vi "UI-BaseParamSet - 副本.vi"(8 "error in (no error)":errorcluster caption="错误输入（无错误）") -> (0 "error out":errorcluster caption="错误输出")   [LabVIEW 2017]
uses:
  Picture/SaveButtom.ctl
  Global System.vi
panel:
  in  "实际孔径":dbl
  in  "Program Update":bool
  in  "Machine Paramter Save Buttom":T1
  out "system time":string
  in  "选项卡控件":enum32{"BaseParamSet", "OtherParamSet"}(tab)
  in  "条码扫描周期":string
  in  "OUT Stack Weigh DataBits":string
  in  "OUT Stack Weigh BaudRate":string
  in  "OUT Stack Weigh VISA Name":refnum<visa-resource-name>="COM1"
  in  "OUT Stack Barcode DataBits":string
  in  "OUT Stack Barcode BaudRate":string
  in  "OUT Stack Barcode VISA Name":refnum<visa-resource-name>="COM1"
  in  "IN Stack Weigh DataBits":string
  in  "IN Stack Weigh BaudRate":string
  in  "IN Stack Weigh VISA Name":refnum<visa-resource-name>="COM1"
  in  "IN Stack Barcode DataBits":string
  in  "IN Stack Barcode BaudRate":string
  in  "IN Stack Barcode VISA Name":refnum<visa-resource-name>="COM1"
  in  "LoadProgram":string(combo)
  in  "BaseParams Save Buttom":T1
  in  "参数B":string
  in  "参数K":string
  in  "校正像素值":string
  in  "Tolerance Params Save":T1
  in  "单位距离":string
  # "秒"
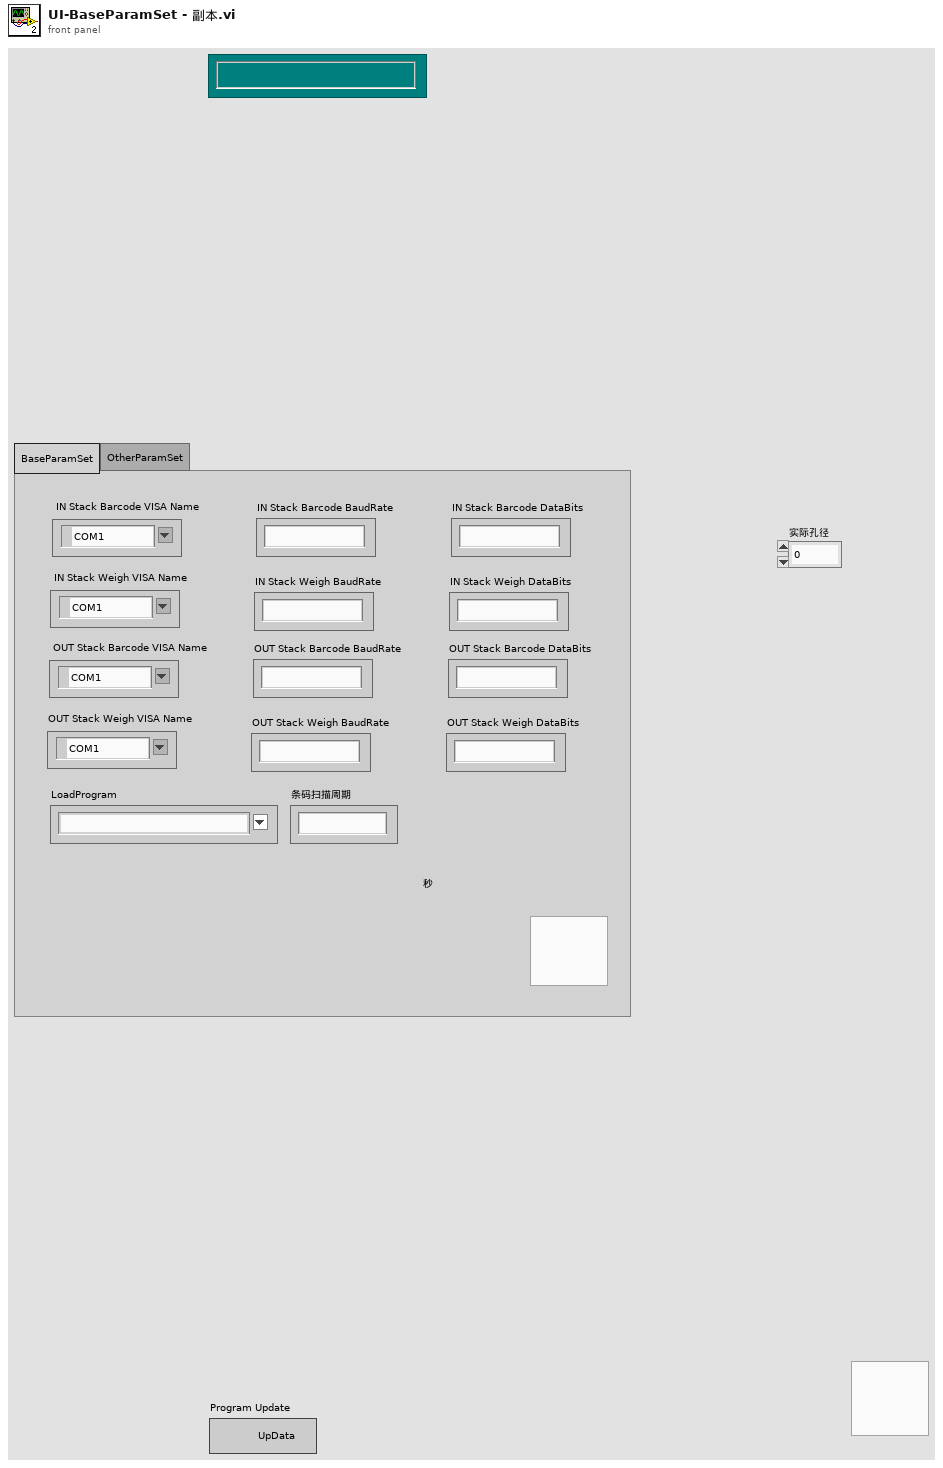
[diagram p1: front panel]
types:
  T1 = typedef "SaveButtom.ctl" = bool
  T2 = cluster{"master data":string, "priority":u16, "secondary data":string[]}
  T3 = cluster{"case name":string[], "queue array":refnum<queue>[]}
  T4 = cluster{"导通气缸上位置":bool, "导通气缸下位置\n":bool, "工位一料到位信号":bool, "工位二料到位信号":bool, "工位三料到位信号":bool, "转盘到位信号":bool, "凸轮感应信号":bool, "导通信号":bool, "真空":bool, "备用":bool, "备用":bool, "备用":bool, "备用":bool, "备用":bool, "备用":bool, "备用":bool, "备用":bool, "备用":bool, "备用":bool, "备用":bool, "备用":bool, "备用":bool, "备用":bool, "备用":bool}
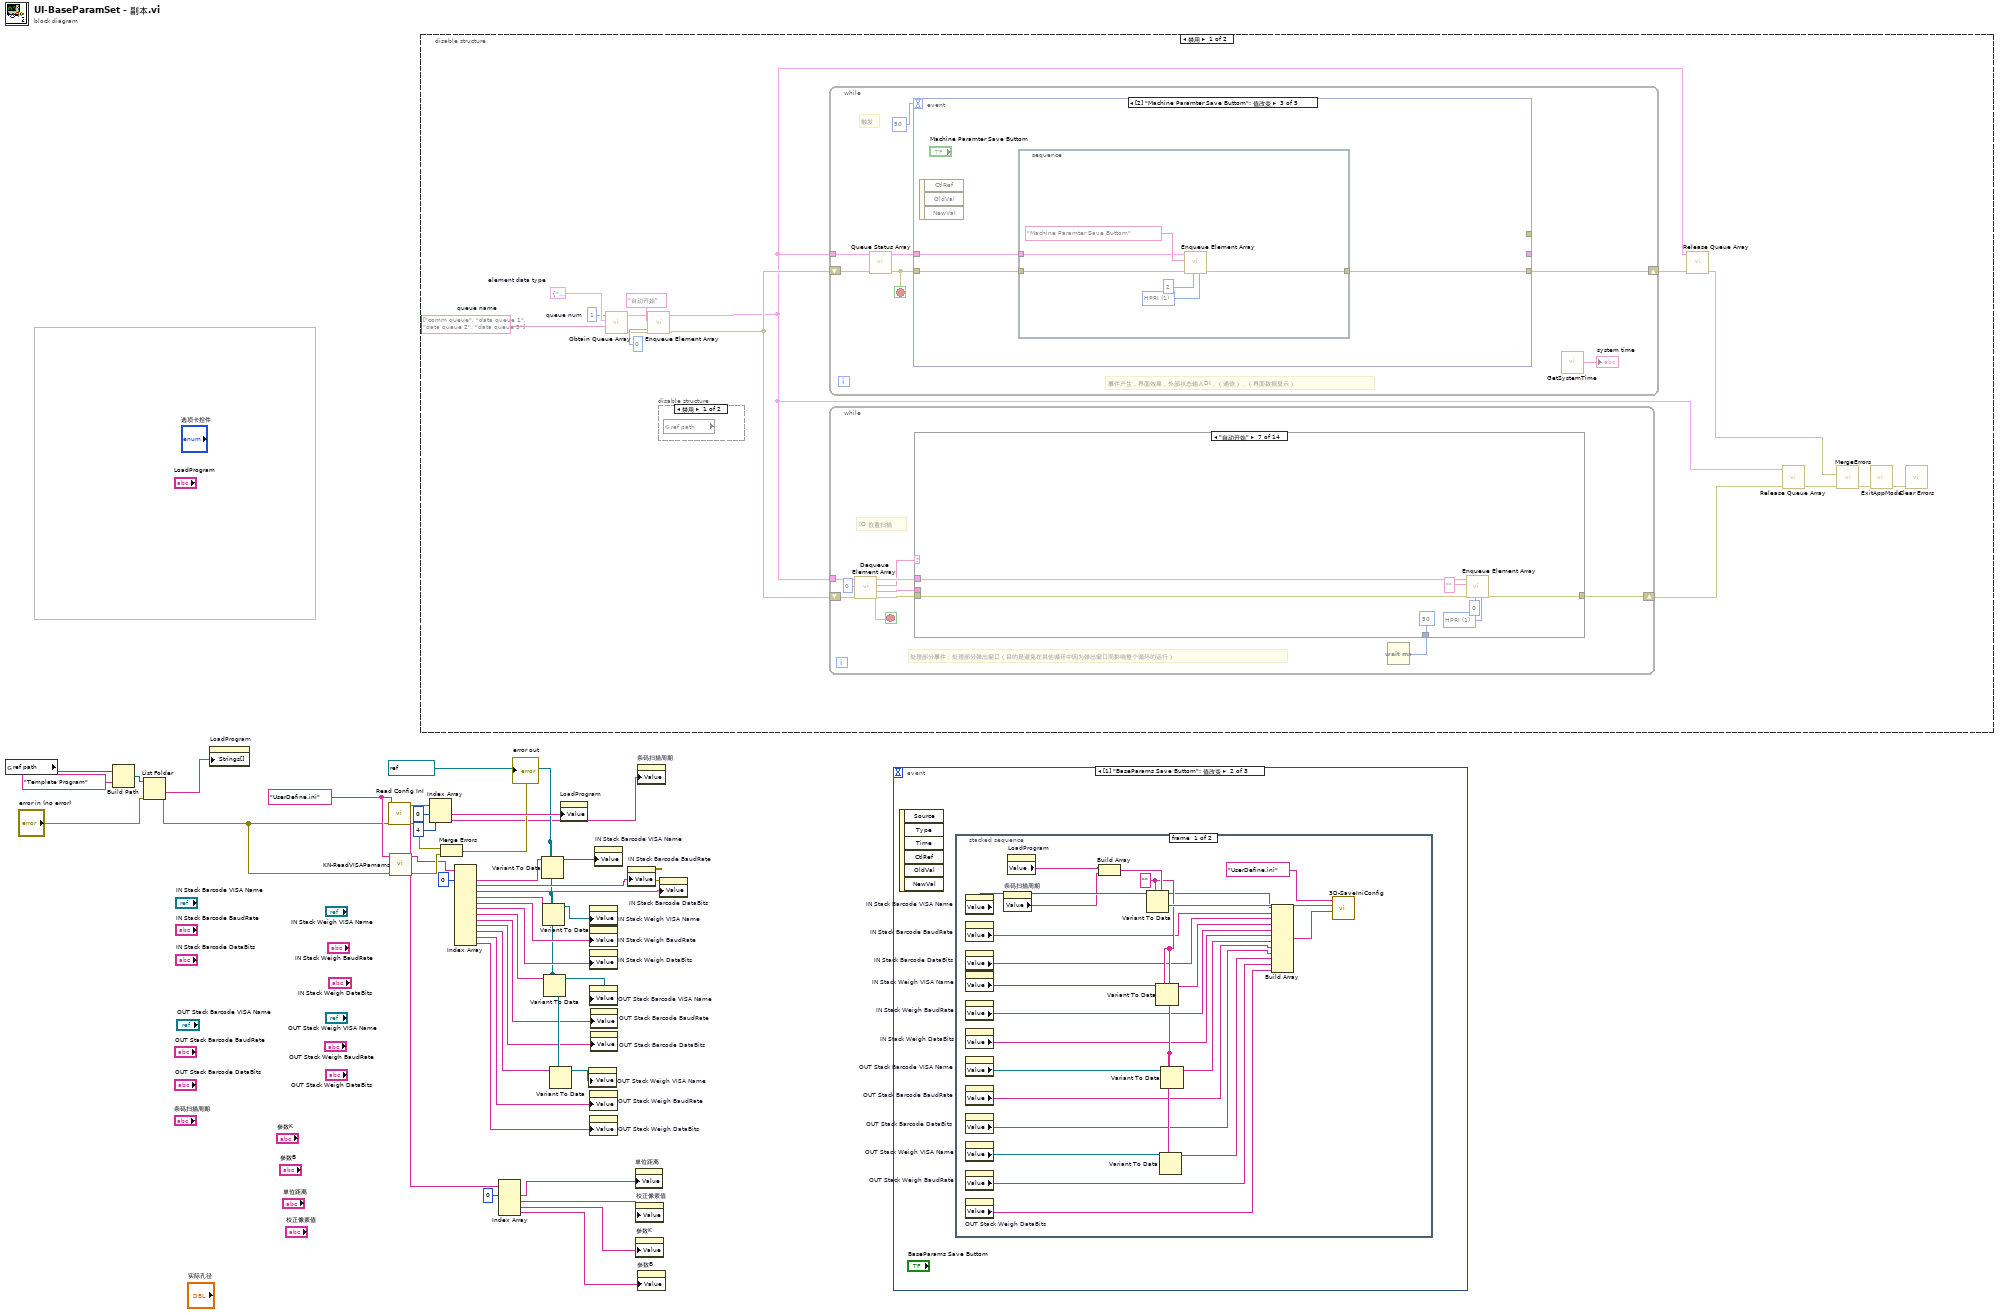
[diagram p0: block diagram]
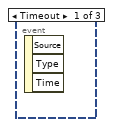
[diagram p2: hidden frame]
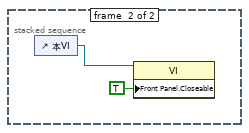
[diagram p3: hidden frame]
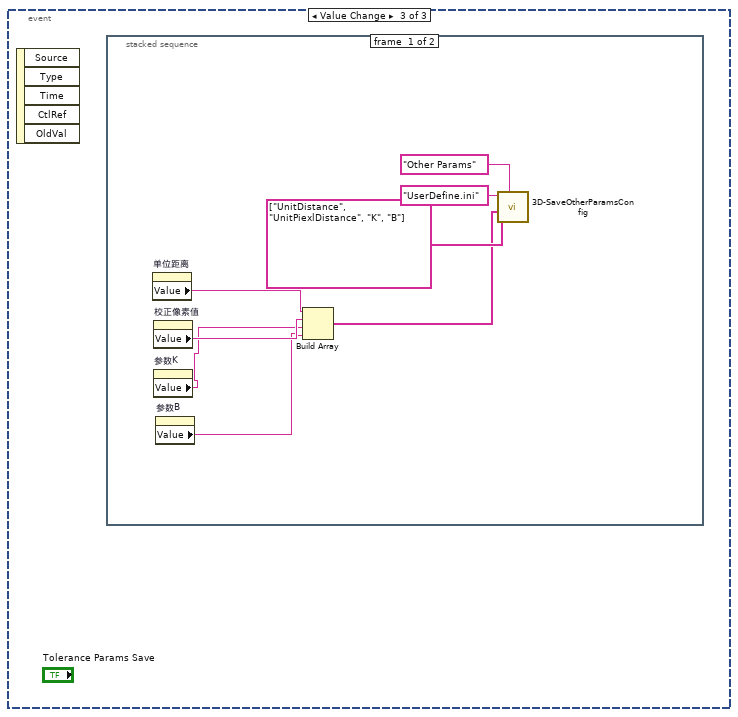
[diagram p4: hidden frame]
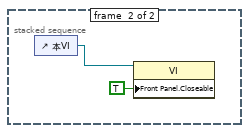
[diagram p5: hidden frame]
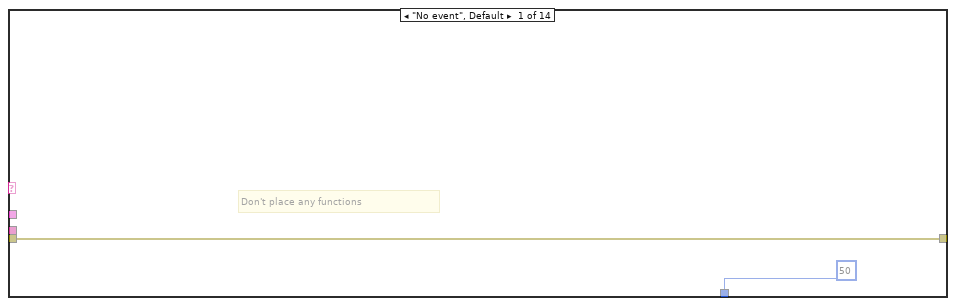
[diagram p7: hidden frame]
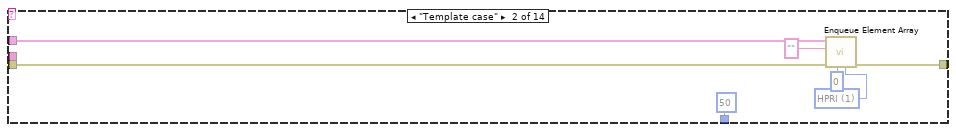
[diagram p8: hidden frame]
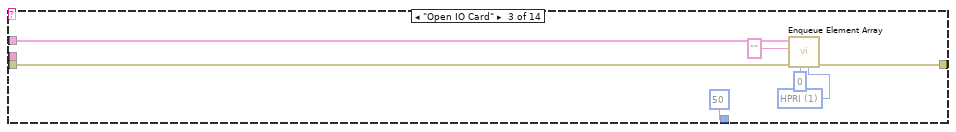
[diagram p9: hidden frame]
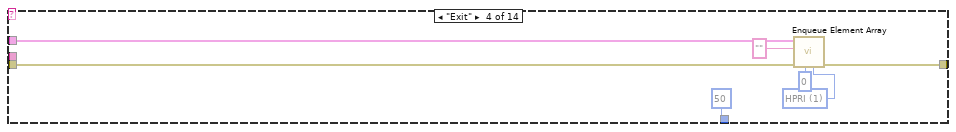
[diagram p10: hidden frame]
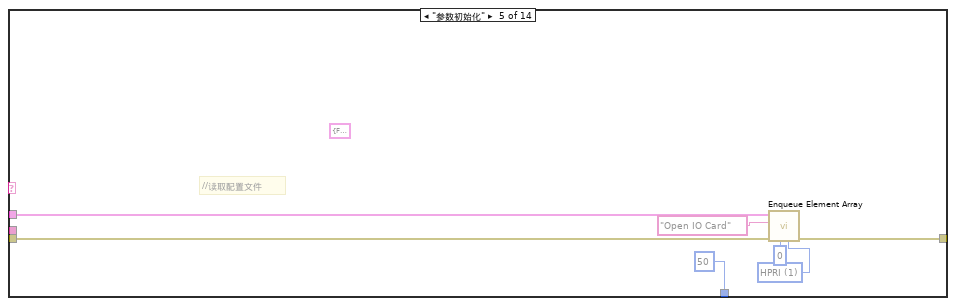
[diagram p11: hidden frame]
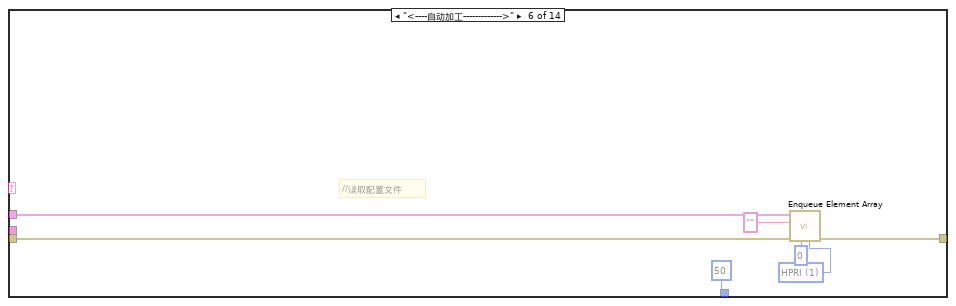
[diagram p12: hidden frame]
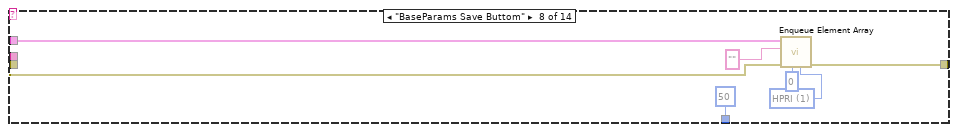
[diagram p13: hidden frame]
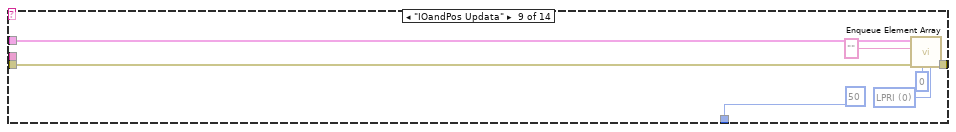
[diagram p14: hidden frame]
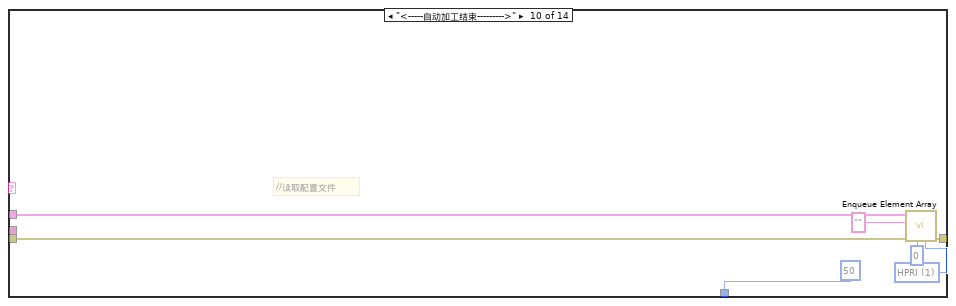
[diagram p15: hidden frame]
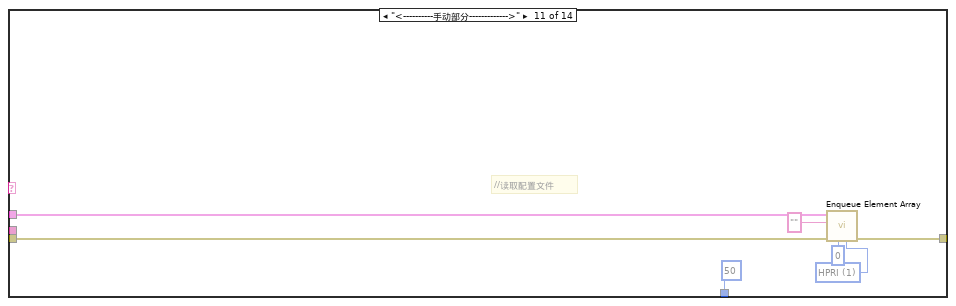
[diagram p16: hidden frame]
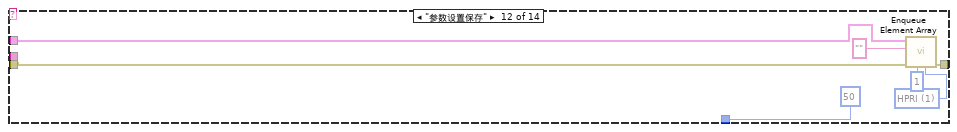
[diagram p17: hidden frame]
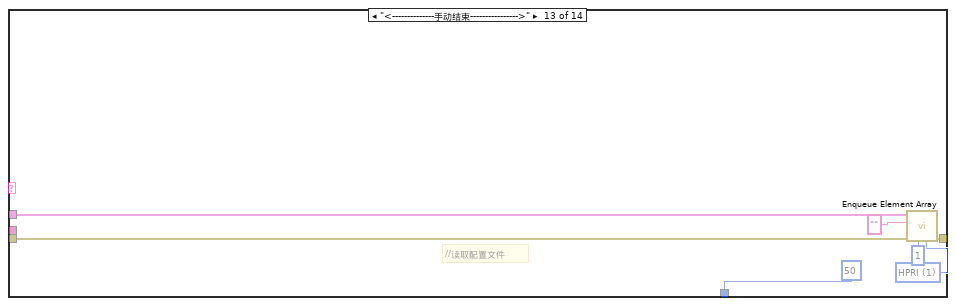
[diagram p18: hidden frame]
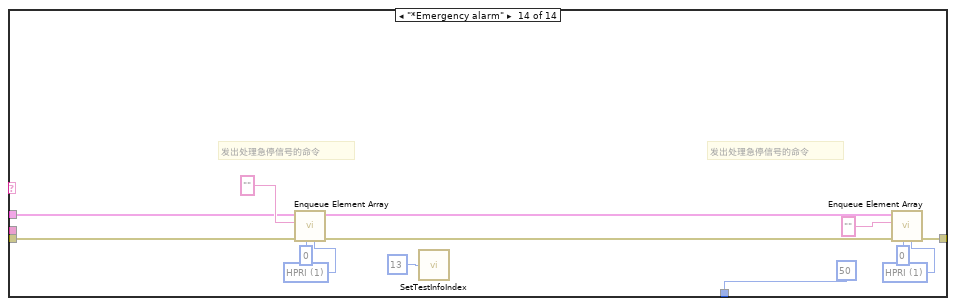
[diagram p19: hidden frame]
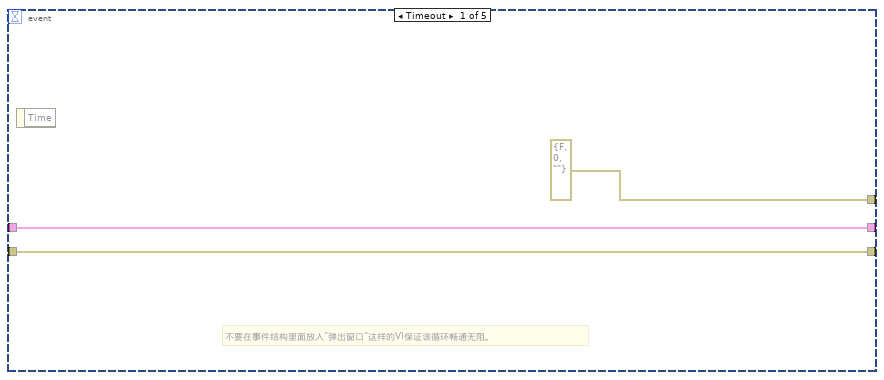
[diagram p20: hidden frame]
diagram:
  w23 = refnum<visa-resource-name> "COM1" ("IN Stack Barcode VISA Name")
  w38 = "UserDefine.ini" ("名称或相对路径")
  n1 = global read "Global System.vi" "ref path"() -> (w14:path)
  n2 = Build Path(base path=w14, name or relative path="Template Program" ("名称或相对路径")) -> (appended path=w12:path)
  n3 = List Folder(path=w12, error in="error in (no error)") -> (folder names=w11:string[], error out=w9:errorcluster)  [unwired: 2 in, 2 out]
  n4 = property on="LoadProgram" class="CmbBox"("Strings[]"=w11) -> ()  [unwired: 2 in, 2 out]
  n5 = call "Read Config InI.vi"("名称或相对路径"=w38, "error in (no error)"=w9) -> ("ParamSet"=w40:string[], "Other Params"=w6:string[], "error out"=w37:errorcluster)  [unwired: 13 in, 2 out]
  n6 = call "KN-ReadVISAPamams.vi"("名称或相对路径"=w38, "error in (no error)"=w9) -> ("VISA1 Param"=w34:string[], "error out"=w36:errorcluster)  [unwired: 12 in]
  n7 = disable-structure shown="禁用" {
    frame Disabled {
      w55 = 1  # queue num
      w56 = T2 {"master data"="", "priority"=0, "secondary data"=[]}  # element data type
      w54 = string[] ["comm queue", "data queue 1", "data queue 2", "data queue 3"]  # queue name
      n8 = call "Obtain Queue Array.vi"("queue name"=w54, "element data type"=w56, "queue num"=w55) -> ("error out"=w50:errorcluster, "queue out"=w51:T3)  [unwired: 2 in, 1 out]
      n9 = call "Enqueue Element Array.vi"("queue index"=0, "error in"=w50, "master data"="自动开始", "queue in"=w51) -> ("error out"=w44:errorcluster, "queue out"=w42:T3)  [unwired: 6 in]
      n10 = disable-structure shown="禁用" {
        frame Disabled {
          n11 = global read "Global System.vi" "ref path"() -> ()  [unwired: 1 out]
        }
        frame Enabled {
        }
      }
      n12 = while {
        shift-right: [w165] -> w45
        shift-left: w44 -> [w168]
        tunnel: w42 -> [w170]
        stop <- w166 stop-if-true
        # "触发"
        # "事件产生，界面效果，外部状态输入DI，（通信），（界面数据显示）"
        n13 = call "Queue Status Array.vi"("error in (no error)"=w168, "queue in"=w170) -> ("error out"=w166:errorcluster, "queue out"=w167:T3)  [unwired: 4 in]
        n14 = event shown="[2] \"Machine Paramter Save Buttom\": 值改变" {
          selector: _ -> [_ _ _ _ _]
          dyn-events: _ -> [_ _ _ _ _]
          timeout: 50 -> [_ _ _ _ _]
          tunnel: [errorcluster {"status"=FALSE, "code"=0, "source"=""} ("error out") _ _ _ _] -> _
          tunnel: w167 -> [w173 w181 w185 w194 w206]
          tunnel: w166 -> [w172 w180 w184 w193 w205]
          tunnel: [w172 w179 w183 w192 w204] -> w165
          tunnel: [w173 w178 _ _ _] -> _
          event Timeout {
            # "不要在事件结构里面放入\"弹出窗口\"这样的VI保证该循环畅通无阻。"
            n15 = event-data() -> ()  [unwired: 1 in, 1 out]
          }
          event Panel Close? {
            w176 = u16 1 items=["HPRI"=1, "LPRI"=0] ("priority")
            n16 = event-data() -> ()  [unwired: 1 in, 4 out]
            n17 = call "Enqueue Element Array.vi"("priority"=w176, "queue index"=0, "error in"=w180, "master data"="*Exit application", "queue in"=w181) -> ("error out"=w179:errorcluster, "queue out"=w178:T3)  [unwired: 5 in]
            n18 = event-data("Discard?"=TRUE) -> ()  [unwired: 1 in, 1 out]
          }
          event Value Change {
            n19 = event-data() -> ()  [unwired: 1 in, 3 out]
            n20 = stacked-sequence {
              tunnel: w185 -> [w188]
              tunnel: w184 -> [w187]
              tunnel: [w186] -> w183
              frame #0 {
                w190 = u16 1 items=["HPRI"=1, "LPRI"=0] ("priority")
                n21 = call "Enqueue Element Array.vi"("priority"=w190, "queue index"=2, "error in"=w187, "master data"="Machine Paramter Save Buttom", "queue in"=w188) -> ("error out"=w186:errorcluster)  [unwired: 5 in, 1 out]
              }
            }
          }
          event "Program Update": Value Change {
            n22 = event-data() -> ()  [unwired: 1 in, 6 out]
            n23 = stacked-sequence {
              tunnel: w194 -> [w197]
              tunnel: w193 -> [w196]
              tunnel: [w195] -> w192
              frame #0 {
                w199 = u16 1 items=["HPRI"=1, "LPRI"=0] ("priority")
                n24 = call "Enqueue Element Array.vi"("priority"=w199, "queue index"=2, "error in"=w196, "master data"="Program Update", "queue in"=w197) -> ("error out"=w195:errorcluster)  [unwired: 5 in, 1 out]
              }
            }
          }
          event Value Change {
            w202 = u16 1 items=["HPRI"=1, "LPRI"=0] ("priority")
            n25 = event-data() -> ()  [unwired: 1 in, 3 out]
            n26 = call "Enqueue Element Array.vi"("priority"=w202, "queue index"=0, "error in"=w205, "master data"="BaseParams Save Buttom", "queue in"=w206) -> ("error out"=w204:errorcluster)  [unwired: 5 in, 1 out]
          }
        }
        n27 = call "GetSystemTime.vi"() -> ("date/time string"=→"system time":string)  [unwired: 7 in]
      }
      n28 = while {
        shift-right: [w65] -> w43
        shift-left: w44 -> [w63]
        tunnel: w42 -> [w59]
        stop <- w58 stop-if-true
        # "IO 位置扫描"
        # "处理部分事件；处理部分弹出窗口（目的是避免在其他循环中因为弹出窗口而影响整个循环的运行）"
        n29 = call "Dequeue Element Array.vi"("queue in"=w59, "queue index"=0, "error in"=w63) -> ("queue out"=w62:T3, "master data"=w61:string, "secondary data"=w60:string[], "error out"=w58:errorcluster)  [unwired: 2 in, 1 out]
        n30 = case shown="\"自动开始\"" w61 {
          tunnel: w62 -> [_ w73 w80 w87 w94 w101 w103 w115 w122 w129 w136 w143 w150 w156]
          tunnel: w58 -> [w67 w70 w77 w84 w91 w98 w106 w112 w117 w126 w133 w140 w147 w153]
          tunnel: [w67 w72 w79 w86 w93 w100 w108 w114 w121 w128 w135 w142 w149 w163] -> w65
          tunnel: [50 50 50 50 50 50 50 50 50 50 50 50 50 50] -> w64
          tunnel: w60 -> [_ _ _ _ _ _ _ _ _ _ _ _ _ _]
          frame "No event", Default {
            # "Don't place any functions"
          }
          frame "Template case" {
            w68 = u16 1 items=["HPRI"=1, "LPRI"=0] ("priority")
            n31 = call "Enqueue Element Array.vi"("priority"=w68, "queue index"=0, "error in"=w70, "master data"="" ("Element 1"), "queue in"=w73) -> ("error out"=w72:errorcluster)  [unwired: 5 in, 1 out]
          }
          frame "Open IO Card" {
            w75 = u16 1 items=["HPRI"=1, "LPRI"=0] ("priority")
            n32 = call "Enqueue Element Array.vi"("priority"=w75, "queue index"=0, "error in"=w77, "master data"="" ("Element 1"), "queue in"=w80) -> ("error out"=w79:errorcluster)  [unwired: 5 in, 1 out]
          }
          frame "Exit" {
            w82 = u16 1 items=["HPRI"=1, "LPRI"=0] ("priority")
            n33 = call "Enqueue Element Array.vi"("priority"=w82, "queue index"=0, "error in"=w84, "master data"="" ("Element 1"), "queue in"=w87) -> ("error out"=w86:errorcluster)  [unwired: 5 in, 1 out]
          }
          frame "参数初始化" {
            (unwired) T4 {"导通气缸上位置"=FALSE, "导通气缸下位置\n"=FALSE, "工位一料到位信号"=FALSE, "工位二料到位信号"=FALSE, "工位三料到位信号"=FALSE, "转盘到位信号"=FALSE, "凸轮感应信号"=FALSE, "导通信号"=FALSE, "真空"=FALSE, "备用"=FALSE, "备用"=FALSE, "备用"=FALSE, "备用"=FALSE, "备用"=FALSE, "备用"=FALSE, "备用"=FALSE, "备用"=FALSE, "备用"=FALSE, "备用"=FALSE, "备用"=FALSE, "备用"=FALSE, "备用"=FALSE, "备用"=FALSE, "备用"=FALSE} ("7230 设备DO")
            w89 = u16 1 items=["HPRI"=1, "LPRI"=0] ("priority")
            # "//读取配置文件"
            n34 = call "Enqueue Element Array.vi"("priority"=w89, "queue index"=0, "error in"=w91, "master data"="Open IO Card" ("Element 1"), "queue in"=w94) -> ("error out"=w93:errorcluster)  [unwired: 5 in, 1 out]
          }
          frame "<----自动加工------------->" {
            w96 = u16 1 items=["HPRI"=1, "LPRI"=0] ("priority")
            # "//读取配置文件"
            n35 = call "Enqueue Element Array.vi"("priority"=w96, "queue index"=0, "error in"=w98, "master data"="" ("Element 1"), "queue in"=w101) -> ("error out"=w100:errorcluster)  [unwired: 5 in, 1 out]
          }
          frame "自动开始" {
            w104 = u16 1 items=["HPRI"=1, "LPRI"=0] ("priority")
            n36 = call "Enqueue Element Array.vi"("priority"=w104, "queue index"=0, "error in"=w106, "master data"="" ("Element 1"), "queue in"=w103) -> ("error out"=w108:errorcluster)  [unwired: 5 in, 1 out]
          }
          frame "BaseParams Save Buttom" {
            w110 = u16 1 items=["HPRI"=1, "LPRI"=0] ("priority")
            n37 = call "Enqueue Element Array.vi"("priority"=w110, "queue index"=0, "error in"=w112, "master data"="" ("Element 1"), "queue in"=w115) -> ("error out"=w114:errorcluster)  [unwired: 5 in, 1 out]
          }
          frame "IOandPos Updata" {
            w119 = u16 0 items=["HPRI"=1, "LPRI"=0] ("priority")
            n38 = call "Enqueue Element Array.vi"("priority"=w119, "queue index"=0, "error in"=w117, "master data"="", "queue in"=w122) -> ("error out"=w121:errorcluster)  [unwired: 5 in, 1 out]
          }
          frame "<-----自动加工结束--------->" {
            w124 = u16 1 items=["HPRI"=1, "LPRI"=0] ("priority")
            # "//读取配置文件"
            n39 = call "Enqueue Element Array.vi"("priority"=w124, "queue index"=0, "error in"=w126, "master data"="" ("Element 1"), "queue in"=w129) -> ("error out"=w128:errorcluster)  [unwired: 5 in, 1 out]
          }
          frame "<----------手动部分------------->" {
            w131 = u16 1 items=["HPRI"=1, "LPRI"=0] ("priority")
            # "//读取配置文件"
            n40 = call "Enqueue Element Array.vi"("priority"=w131, "queue index"=0, "error in"=w133, "master data"="" ("Element 1"), "queue in"=w136) -> ("error out"=w135:errorcluster)  [unwired: 5 in, 1 out]
          }
          frame "参数设置保存" {
            w138 = u16 1 items=["HPRI"=1, "LPRI"=0] ("priority")
            n41 = call "Enqueue Element Array.vi"("priority"=w138, "queue index"=1, "error in"=w140, "master data"="" ("Element 1"), "queue in"=w143) -> ("error out"=w142:errorcluster)  [unwired: 5 in, 1 out]
          }
          frame "<--------------手动结束---------------->" {
            w145 = u16 1 items=["HPRI"=1, "LPRI"=0] ("priority")
            # "//读取配置文件"
            n42 = call "Enqueue Element Array.vi"("priority"=w145, "queue index"=1, "error in"=w147, "master data"="" ("Element 1"), "queue in"=w150) -> ("error out"=w149:errorcluster)  [unwired: 5 in, 1 out]
          }
          frame "*Emergency alarm" {
            w159 = u16 1 items=["HPRI"=1, "LPRI"=0] ("priority")
            w160 = u16 1 items=["HPRI"=1, "LPRI"=0] ("priority")
            # "发出处理急停信号的命令"
            # "发出处理急停信号的命令"
            n43 = call "Enqueue Element Array.vi"("priority"=w159, "queue index"=0, "error in"=w153, "master data"="" ("Element 1"), "queue in"=w156) -> ("error out"=w154:errorcluster, "queue out"=w155:T3)  [unwired: 5 in]
            n44 = call "SetTestInfoIndex.vi"("test info index"=13) -> ()
            n45 = call "Enqueue Element Array.vi"("priority"=w160, "queue index"=0, "error in"=w154, "master data"="" ("Element 1"), "queue in"=w155) -> ("error out"=w163:errorcluster)  [unwired: 5 in, 1 out]
          }
        }
        n46 = Wait (ms)(milliseconds to wait=w64) -> ()  [unwired: 1 out]
      }
      n47 = call "Release Queue Array.vi"("error in"=w45, "queue in"=w42) -> ("error out"=w47:errorcluster)  [unwired: 2 in, 3 out]
      n48 = call "Release Queue Array.vi"("error in"=w43, "queue in"=w42) -> ("error out"=w49:errorcluster)  [unwired: 2 in, 3 out]
      n49 = call "MergeErrors.vi"("error in 2 (no error)"=w47, "error in 4 (no error)"=w49) -> ("error out"=w48:errorcluster)  [unwired: 6 in]
      n50 = call "ExitAppMode.vi"("error in (no error)"=w48) -> ("error out"=w46:errorcluster)  [unwired: 10 in]
      n51 = call <vilib>:"Clear Errors.vi"("error in (no error)"=w46) -> ()  [unwired: 5 in, 2 out]
    }
    frame Enabled {
    }
  }
  n52 = Index Array(array=w40, index #1=0 ("索引"), index #2=4 ("索引")) -> (element #1=w39:string, element #2=w7:string)
  n53 = Merge Errors(w37, w36) -> (→"error out":errorcluster)
  n54 = Index Array(array=w34, index #1=0 ("索引")) -> (element #1=w32:string, element #2=w30:string, element #3=w28:string, element #4=w27:string, element #5=w25:string, element #6=w24:string, element #7=w22:string, element #8=w20:string, element #9=w19:string, element #10=w18:string, element #11=w16:string, element #12=w15:string)  [unwired: 11 in]
  n55 = Index Array(array=w6, index #1=0 ("索引")) -> (element #1=w4:string, element #2=w3:string, element #3=w2:string, element #4=w1:string)  [unwired: 3 in]
  n56 = Variant To Data(type=w23, Variant=w32) -> (data=w31:refnum<visa-resource-name>)  [unwired: 1 in, 1 out]
  n57 = Variant To Data(type=w23, Variant=w27) -> (data=w26:refnum<visa-resource-name>)  [unwired: 1 in, 1 out]
  n58 = Variant To Data(type=w23, Variant=w22) -> (data=w21:refnum<visa-resource-name>)  [unwired: 1 in, 1 out]
  n59 = Variant To Data(type=w23, Variant=w18) -> (data=w17:refnum<visa-resource-name>)  [unwired: 1 in, 1 out]
  n60 = property on="LoadProgram" class="CmbBox"("Value"=w39) -> ()  [unwired: 2 in, 2 out]
  n61 = property on="OUT Stack Weigh VISA Name" class="VISAName"("Value"=w17) -> ()  [unwired: 2 in, 2 out]
  n62 = property on="IN Stack Weigh VISA Name" class="VISAName"("Value"=w26) -> ()  [unwired: 2 in, 2 out]
  n63 = property on="IN Stack Weigh BaudRate" class="Str"("Value"=w25) -> ()  [unwired: 2 in, 2 out]
  n64 = property on="IN Stack Weigh DataBits" class="Str"("Value"=w24) -> ()  [unwired: 2 in, 2 out]
  n65 = property on="OUT Stack Barcode VISA Name" class="VISAName"("Value"=w21) -> ()  [unwired: 2 in, 2 out]
  n66 = property on="OUT Stack Weigh BaudRate" class="Str"("Value"=w16) -> ()  [unwired: 2 in, 2 out]
  n67 = property on="OUT Stack Weigh DataBits" class="Str"("Value"=w15) -> ()  [unwired: 2 in, 2 out]
  n68 = property on="OUT Stack Barcode BaudRate" class="Str"("Value"=w20) -> ()  [unwired: 2 in, 2 out]
  n69 = property on="OUT Stack Barcode DataBits" class="Str"("Value"=w19) -> ()  [unwired: 2 in, 2 out]
  n70 = property on="IN Stack Barcode VISA Name" class="VISAName"("Value"=w31) -> ()  [unwired: 2 in, 2 out]
  n71 = property on="IN Stack Barcode BaudRate" class="Str"("Value"=w30) -> (error out=w29:errorcluster)  [unwired: 2 in, 1 out]
  n72 = property on="单位距离" class="Str"("Value"=w4) -> ()  [unwired: 2 in, 2 out]
  n73 = property on="校正像素值" class="Str"("Value"=w3) -> ()  [unwired: 2 in, 2 out]
  n74 = property on="参数K" class="Str"("Value"=w2) -> ()  [unwired: 2 in, 2 out]
  n75 = property on="条码扫描周期" class="Str"("Value"=w7) -> ()  [unwired: 2 in, 2 out]
  n76 = property on="参数B" class="Str"("Value"=w1) -> ()  [unwired: 2 in, 2 out]
  n77 = property on="IN Stack Barcode DataBits" class="Str"(error in=w29, "Value"=w28) -> ()  [unwired: 1 in, 2 out]
  n78 = event shown="[1] \"BaseParams Save Buttom\": 值改变" {
    selector: _ -> [_ _ _]
    dyn-events: _ -> [_ _ _]
    timeout: _ -> [_ _ _]
    event Timeout {
      n79 = event-data() -> ()  [unwired: 1 in, 3 out]
    }
    event Value Change {
      n80 = event-data() -> ()  [unwired: 1 in, 6 out]
      n81 = stacked-sequence {
        frame #0 {
          w224 = ""
          n82 = property on="IN Stack Barcode VISA Name" class="VISAName"() -> ("Value"=w225:refnum<visa-resource-name>)  [unwired: 2 in, 2 out]
          n83 = property on="IN Stack Barcode BaudRate" class="Str"() -> ("Value"=w219:string)  [unwired: 2 in, 2 out]
          n84 = property on="IN Stack Barcode DataBits" class="Str"() -> ("Value"=w218:string)  [unwired: 2 in, 2 out]
          n85 = property on="IN Stack Weigh VISA Name" class="VISAName"() -> ("Value"=w223:refnum<visa-resource-name>)  [unwired: 2 in, 2 out]
          n86 = property on="IN Stack Weigh BaudRate" class="Str"() -> ("Value"=w216:string)  [unwired: 2 in, 2 out]
          n87 = property on="IN Stack Weigh DataBits" class="Str"() -> ("Value"=w215:string)  [unwired: 2 in, 2 out]
          n88 = property on="OUT Stack Barcode VISA Name" class="VISAName"() -> ("Value"=w222:refnum<visa-resource-name>)  [unwired: 2 in, 2 out]
          n89 = property on="OUT Stack Barcode BaudRate" class="Str"() -> ("Value"=w213:string)  [unwired: 2 in, 2 out]
          n90 = property on="OUT Stack Barcode DataBits" class="Str"() -> ("Value"=w212:string)  [unwired: 2 in, 2 out]
          n91 = property on="OUT Stack Weigh VISA Name" class="VISAName"() -> ("Value"=w221:refnum<visa-resource-name>)  [unwired: 2 in, 2 out]
          n92 = property on="OUT Stack Weigh BaudRate" class="Str"() -> ("Value"=w210:string)  [unwired: 2 in, 2 out]
          n93 = property on="OUT Stack Weigh DataBits" class="Str"() -> ("Value"=w209:string)  [unwired: 2 in, 2 out]
          n94 = property on="条码扫描周期" class="Str"() -> ("Value"=w207:string)  [unwired: 2 in, 2 out]
          n95 = property on="LoadProgram" class="CmbBox"() -> ("Value"=w227:string)  [unwired: 2 in, 2 out]
          n96 = Build Array(w227, w207) -> (w226:string[])
          n97 = Variant To Data(type=w224, Variant=w225) -> (data=w220:string)  [unwired: 1 in, 1 out]
          n98 = Variant To Data(type=w224, Variant=w223) -> (data=w217:string)  [unwired: 1 in, 1 out]
          n99 = Variant To Data(type=w224, Variant=w221) -> (data=w211:string)  [unwired: 1 in, 1 out]
          n100 = Variant To Data(type=w224, Variant=w222) -> (data=w214:string)  [unwired: 1 in, 1 out]
          n101 = Build Array(w220, w219, w218, w217, w216, w215, w214, w213, w212, w211, w210, w209) -> (w208:string[])
          n102 = call "3D-SaveIniConfig.vi"("VISA1"=w208, "Inputs_BaseParam"=w226, "名称或相对路径"="UserDefine.ini") -> ()  [unwired: 9 in]
        }
        frame #1 {
          n103 = control-ref of="本VI"() -> (w230:refnum<vi>)
          n104 = property class="VI"(reference=w230, "Front Panel.Closeable"=TRUE ("前面板窗口:可关闭")) -> ()  [unwired: 1 in, 2 out]
        }
      }
    }
    event Value Change {
      n105 = event-data() -> ()  [unwired: 1 in, 5 out]
      n106 = stacked-sequence {
        frame #0 {
          n107 = property on="单位距离" class="Str"() -> ("Value"=w235:string)  [unwired: 2 in, 2 out]
          n108 = property on="校正像素值" class="Str"() -> ("Value"=w234:string)  [unwired: 2 in, 2 out]
          n109 = property on="参数K" class="Str"() -> ("Value"=w233:string)  [unwired: 2 in, 2 out]
          n110 = property on="参数B" class="Str"() -> ("Value"=w232:string)  [unwired: 2 in, 2 out]
          n111 = Build Array(w235, w234, w233, w232) -> (w231:string[])
          n112 = call "3D-SaveOtherParamsConfig.vi"("section"="Other Params", "Values"=w231, "Keys"=string[] ["UnitDistance", "UnitPiexlDistance", "K", "B"], "名称或相对路径"="UserDefine.ini") -> ()  [unwired: 8 in]
        }
        frame #1 {
          n113 = control-ref of="本VI"() -> (w240:refnum<vi>)
          n114 = property class="VI"(reference=w240, "Front Panel.Closeable"=TRUE ("前面板窗口:可关闭")) -> ()  [unwired: 1 in, 2 out]
        }
      }
    }
  }
